vi "Tree_Get first enabled element from top.vi"(8 "error in (no error)":errorcluster, 11 "Tree Control Ref":refnum<vi>) -> (0 "error out":errorcluster, 2 "First Enabled Element":string, 3 "Tree Control Ref Out":refnum<vi>)   [LabVIEW 2023]
panel:
  in  "Tree":string[](tree)
  # "DEBUG"
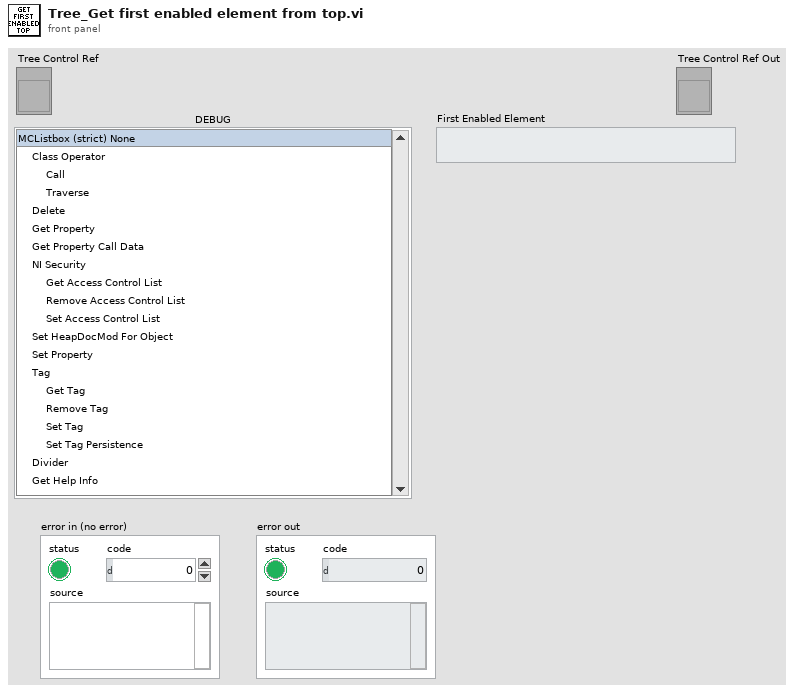
[diagram p1: front panel]
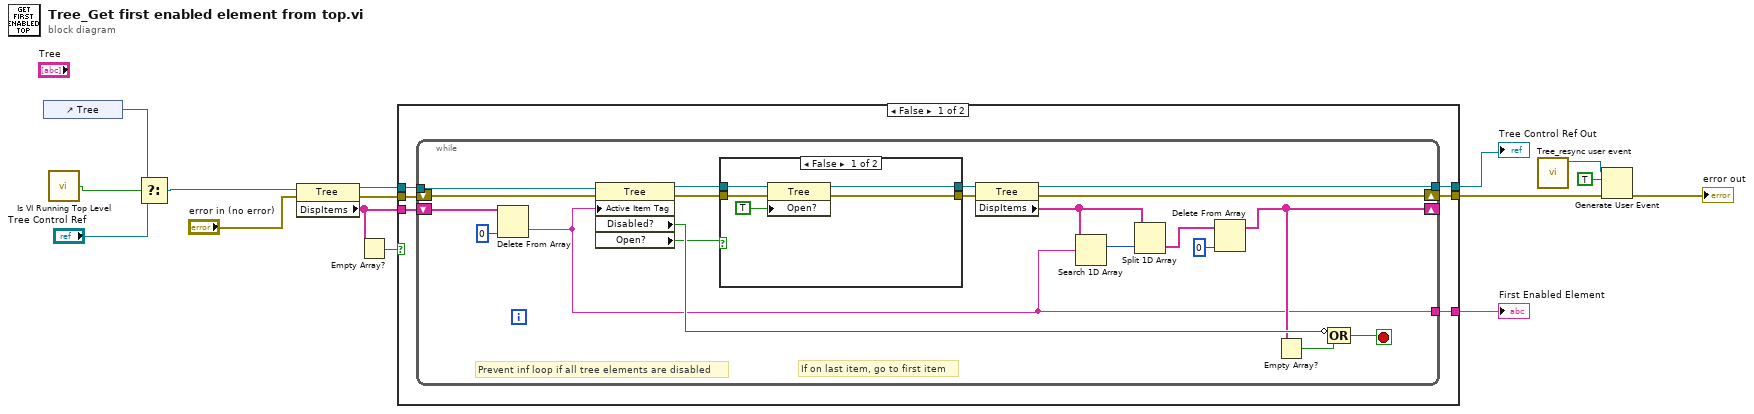
[diagram p0: block diagram]
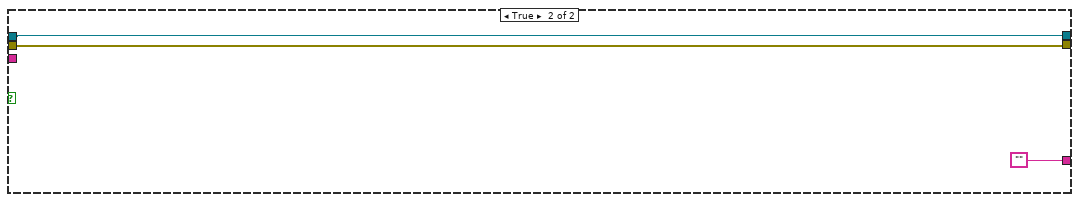
[diagram p3: hidden frame]
diagram:
  n1 = control-ref of="Tree"() -> (w11:refnum<vi>)
  n2 = call "Is VI Running Top Level.vi"() -> ("Top Level?"=w12:bool)  [unwired: 5 in]
  n3 = Select(t=w11, s=w12, f="Tree Control Ref") -> (s? t:f=w9:refnum<vi>)
  n4 = property class="Tree"(reference=w9, error in="error in (no error)") -> (reference out=w14:refnum<vi>, error out=w13:errorcluster, "DispItems"=w2:string[])
  n5 = Empty Array?(array=w2) -> (empty?=w1:bool)
  n6 = case shown="False" w1 {
    tunnel: w14 -> [w21 w50]
    tunnel: w13 -> [w20 w51]
    tunnel: w2 -> [w19 _]
    tunnel: [w18 ""] -> w8
    tunnel: [w17 w50] -> w7
    tunnel: [w16 w51] -> w4
    frame False {
      n7 = while {
        tunnel: w21 -> [w38]
        shift-right: [w35] -> w16
        shift-left: w20 -> [w34]
        shift-right: [w26] -> _
        shift-left: w19 -> [w36]
        tunnel: [w25] -> w18
        tunnel: [w24] -> w17
        stop <- w32 stop-if-true
        # "Prevent inf loop if all tree elements are disabled"
        # "If on last item, go to first item"
        n8 = Delete From Array(array=w36, index=0) -> (deleted portion=w25:string)  [unwired: 1 in, 1 out]
        n9 = property class="Tree"(reference=w38, error in=w34, "Active Item Tag"=w25) -> (reference out=w41:refnum<vi>, error out=w39:errorcluster, "Disabled?"=w40:bool, "Open?"=w22:bool)
        n10 = case shown="False" w22 {
          tunnel: w41 -> [w46 w48]
          tunnel: w39 -> [w45 w47]
          tunnel: [w44 w48] -> w31
          tunnel: [w43 w47] -> w23
          frame False {
            n11 = property class="Tree"(reference=w46, error in=w45, "Open?"=TRUE ("Active Item:Open?")) -> (reference out=w44:refnum<vi>, error out=w43:errorcluster)
          }
          frame True {
          }
        }
        n12 = property class="Tree"(reference=w31, error in=w23) -> (reference out=w24:refnum<vi>, error out=w35:errorcluster, "DispItems"=w30:string[])
        n13 = Search 1D Array(1D array=w30, element=w25) -> (index of element=w29:i32)  [unwired: 1 in]
        n14 = Split 1D Array(array=w30, index=w29) -> (second subarray=w28:string[])  [unwired: 1 out]
        n15 = Delete From Array(array=w28, index=0) -> (array with subset deleted=w26:string[])  [unwired: 1 in, 1 out]
        n16 = Empty Array?(array=w26) -> (empty?=w33:bool)
        n17 = Compound Arithmetic op=OR(invert w40, w33) -> (w32:bool)
      }
    }
    frame True {
    }
  }
  "First Enabled Element" <- w8
  "Tree Control Ref Out" <- w7
  n18 = call "Tree_resync user event.vi"() -> ("Open/close"=w6:refnum<user-event>)  [unwired: 11 in]
  n19 = Generate User Event(user event=w6, event data cluster=TRUE ("event data"), error in=w4) -> (error out=→"error out":errorcluster)  [unwired: 1 in, 1 out]
